vi "Advance past Object.vi"(7 "JSON":string, 9 "Offset":i32) -> (1 "Offset past Object":i32, 3 "State":T1, 6 "Object Start":i32)   [LabVIEW 2017, in "JSONtext.lvlib"]
uses:
  JSONtext.lvlib
  Parsing State.ctl
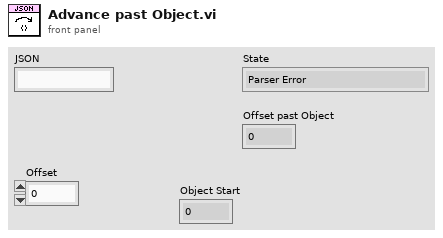
[diagram p1: front panel]
types:
  T1 = typedef "JSONtext.lvlib/Parsing State.ctl" = enum16{"Parser Error", "Object", "Array", "String", "Number/Other", "Leading Whitespace", "Object end", "Array end", "Value end"}
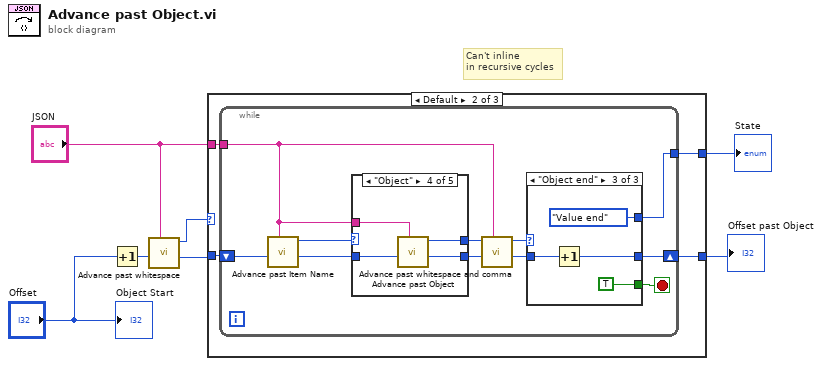
[diagram p0: block diagram]
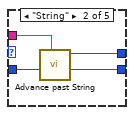
[diagram p4: hidden frame]
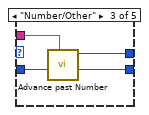
[diagram p5: hidden frame]
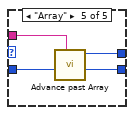
[diagram p6: hidden frame]
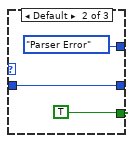
[diagram p8: hidden frame]
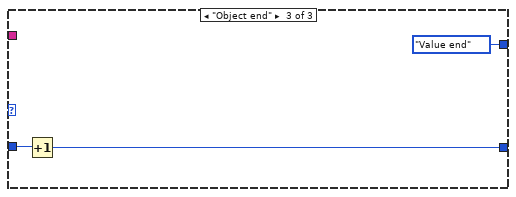
[diagram p9: hidden frame]
diagram:
  # "Can't inline\nin recursive cycles"
  n1 = Increment(x="Offset") -> (x+1=w3:i32)
  n2 = call "Advance past whitespace.vi"("JSON"="JSON", "Offset"=w3) -> ("Offset of first non-whitespace"=w2:i32, "Parser State"=w1:T1)  [unwired: 8 in]
  n3 = case shown="Default" w1 {
    selector: w1 -> [w8 _ _]
    tunnel: [w8 w13 Parsing_State."Value end"] -> w7
    tunnel: [w9 w12 w51] -> w6
    tunnel: w2 -> [w9 w11 w52]
    tunnel: "JSON" -> [_ w10 _]
    frame "Parser Error", "Array end" {
    }
    frame Default {
      n4 = while {
        shift-right: [w22] -> w12
        shift-left: w11 -> [w19]
        tunnel: w10 -> [w16]
        tunnel: [w20] -> w13
        stop <- w21 stop-if-true
        n5 = call "Advance past Item Name.vi"("JSON"=w16, "Offset"=w19) -> ("Offset past colon"=w14:i32, "State"=w15:T1)  [unwired: 6 in, 2 out]
        n6 = case shown="\"Object\"" w15 {
          selector: w15 -> [w26 _ _ _ _]
          tunnel: w14 -> [w25 w30 w34 w38 w42]
          tunnel: [w26 w28 w32 w37 w41] -> w18
          tunnel: [w25 w29 w33 w36 w40] -> w17
          tunnel: w16 -> [_ w27 w31 w35 w39]
          frame Default {
          }
          frame "String" {
            n7 = call "Advance past String.vi"("JSON"=w27, "Offset"=w30) -> ("Offset past match"=w29:i32, "State"=w28:T1)  [unwired: 7 in, 1 out]
          }
          frame "Number/Other" {
            n8 = call "Advance past Number.vi"("JSON"=w31, "Offset (0)"=w34) -> ("Offset past match"=w33:i32, "Parser State"=w32:T1)  [unwired: 6 in, 2 out]
          }
          frame "Object" {
            n9 = call "Advance past Object.vi"("JSON"=w35, "Offset"=w38) -> ("Offset past Object"=w36:i32, "State"=w37:T1)  [unwired: 7 in, 1 out]
          }
          frame "Array" {
            n10 = call "Advance past Array.vi"("JSON"=w39, "Offset"=w42) -> ("Offset past Array"=w40:i32, "State"=w41:T1)  [unwired: 6 in, 2 out]
          }
        }
        n11 = call "Advance past whitespace and comma.vi"("JSON"=w16, "Offset"=w17, "State in"=w18) -> ("Offset past match"=w24:i32, "State"=w23:T1)  [unwired: 7 in]
        n12 = case shown="\"Object end\"" w23 {
          tunnel: [_ TRUE TRUE] -> w21
          tunnel: [_ Parsing_State."Parser Error" Parsing_State."Value end"] -> w20
          tunnel: w24 -> [w43 w44 w48]
          tunnel: [w43 w44 w47] -> w22
          frame "Object".."Number/Other" {
          }
          frame Default {
          }
          frame "Object end" {
            n13 = Increment(x=w48) -> (x+1=w47:i32)
          }
        }
      }
    }
    frame "Object end" {
      n14 = Increment(x=w52) -> (x+1=w51:i32)
    }
  }
  "State" <- w7
  "Offset past Object" <- w6
  "Object Start" <- "Offset"
